vi "AudioMixAnalyzer.vi"() -> ()   [LabVIEW 2014]
panel:
  in  "Output File":path
  in  "Playback":bool
  in  "Record":bool
  in  "stop":bool
  out "Recorded Wave Form":dynamicdata(graph)
  in  "Band-pass Filter":bool
  in  "Lower Cut-off Frequency (Hz)":dbl
  in  "Upper Cut-off Frequency (Hz)":dbl
  # "AudioMixAnalyzer.vi -- Authored: Josh Reyes and Josh Borgman\n\nThis VI allow the user to record audio input and apply a band-pass filter to the recorded audio for real-time manipulation. The recorded audio is then saved to an audio file (.wav) whose file path is designated by the dialouge box below the waveform."
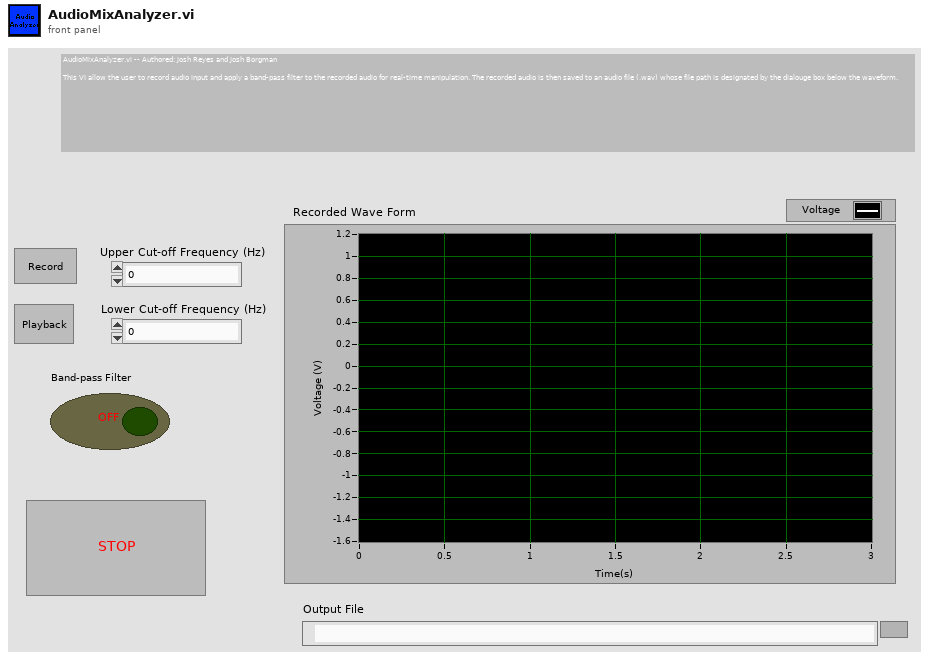
[diagram p1: front panel]
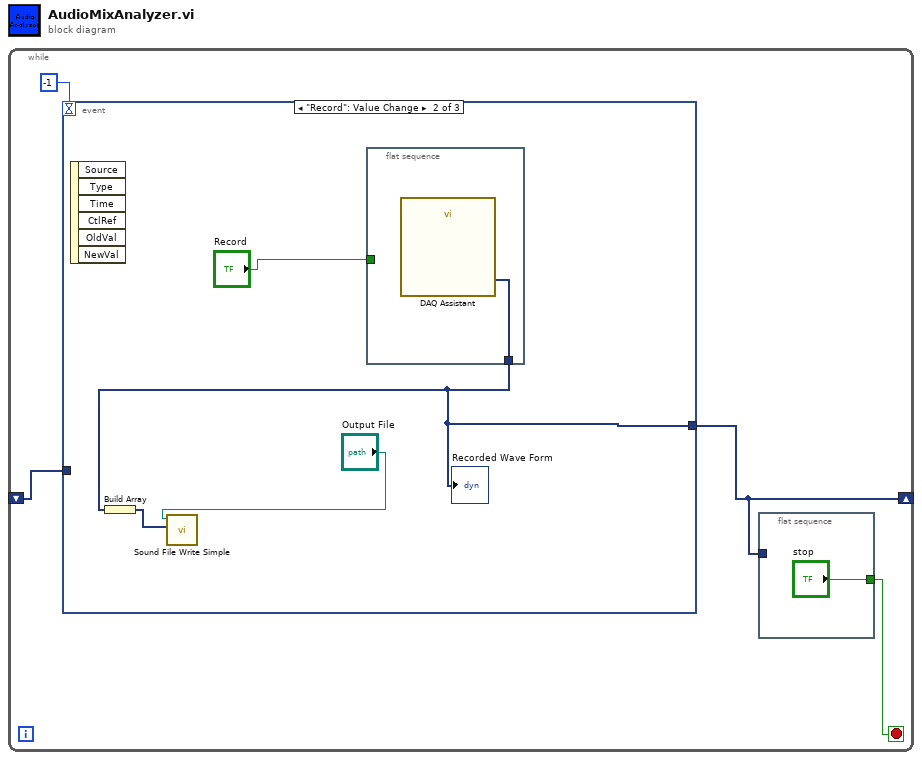
[diagram p0: block diagram]
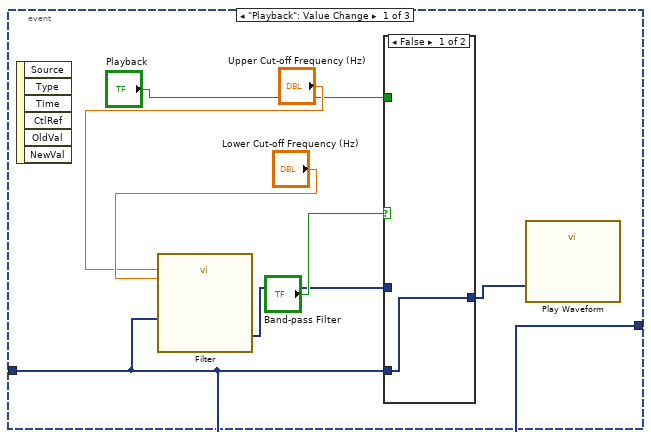
[diagram p2: hidden frame]
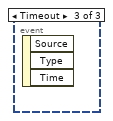
[diagram p4: hidden frame]
diagram:
  n1 = while {
    shift-right: [w3] -> _
    shift-left: _ -> [w1]
    stop <- w2 stop-if-true
    n2 = event shown="[1] \"Record\": Value Change" {
      selector: _ -> [_ _ _]
      dyn-events: _ -> [_ _ _]
      timeout: -1 -> [_ _ _]
      tunnel: [w8 w15 _] -> w3
      tunnel: w1 -> [w8 _ _]
      event "Playback": Value Change {
        n3 = event-data() -> ()  [unwired: 1 in, 6 out]
        n4 = call "Filter"("Lower Cut-Off"="Lower Cut-off Frequency (Hz)", "Upper Cut-Off"="Upper Cut-off Frequency (Hz)", "Signal"=w8) -> ("Filtered Signal"=w9:dynamicdata)  [unwired: 7 in, 1 out]
        n5 = case shown="False" "Band-pass Filter" {
          tunnel: "Playback" -> [_ _]
          tunnel: w9 -> [_ w14]
          tunnel: w8 -> [w13 _]
          tunnel: [w13 w14] -> w7
          frame False {
          }
          frame True {
          }
        }
        n6 = call "Play Waveform"("Data"=w7) -> ()  [unwired: 18 in, 1 out]
      }
      event "Record": Value Change {
        n7 = event-data() -> ()  [unwired: 1 in, 6 out]
        n8 = Build Array(w15) -> (w17:dynamicdata[])
        n9 = call <vilib>:"Sound File Write Simple.vi"("data"=w17, "path"="Output File") -> ()  [unwired: 8 in, 2 out]
        n10 = flat-sequence {
          tunnel: [w19] -> w15
          tunnel: "Record" -> [_]
          frame #0 {
            n11 = call "DAQ Assistant"() -> ("data"=w19:dynamicdata)  [unwired: 16 in, 3 out]
          }
        }
        "Recorded Wave Form" <- w15
      }
      event Timeout {
        n12 = event-data() -> ()  [unwired: 1 in, 3 out]
      }
    }
    n13 = flat-sequence {
      tunnel: w3 -> [_]
      tunnel: ["stop"] -> w2
      frame #0 {
      }
    }
  }
